vi "PCANTerminal1.vi"() -> ()   [LabVIEW 2020]
uses:
  <userlib>/PCAN-Basic/PCANBasic.lvlib
panel:
  out "x-y":u32
  out "function return 4":u32 format="%x"
  out "function return 3":u32 format="%.0x"
  in  "MessageBuffer":T1(array[cluster])=[{"ID"=828, "MSGTYPE"=0, "LEN"=8, "DATA[0]"=2, "DATA[1]"=0, "DATA[2]"=0, "DATA[3]"=0, "DATA[4]"=0, "DATA[5]"=0, "DATA[6]"=0, "DATA[7]"=0}, {"ID"=860, "MSGTYPE"=0, "LEN"=8, "DATA[0]"=20, "DATA[1]"=0, "DATA[2]"=169, "DATA[3]"=128, "DATA[4]"=74, "DATA[5]"=148, "DATA[6]"=160, "DATA[7]"=9}, {"ID"=917, "MSGTYPE"=0, "LEN"=8, "DATA[0]"=0, "DATA[1]"=0, "DATA[2]"=0, "DATA[3]"=0, "DATA[4]"=0, "DATA[5]"=0, "DATA[6]"=0, "DATA[7]"=0}, {"ID"=1409, "MSGTYPE"=0, "LEN"=8, "DATA[0]"=129, "DATA[1]"=0, "DATA[2]"=0, "DATA[3]"=0, "DATA[4]"=0, "DATA[5]"=0, "DATA[6]"=0, "DATA[7]"=0}, {"ID"=911, "MSGTYPE"=0, "LEN"=8, "DATA[0]"=0, "DATA[1]"=0, "DATA[2]"=8, "DATA[3]"=0, "DATA[4]"=0, "DATA[5]"=0, "DATA[6]"=0, "DATA[7]"=0}] {"ID" format="%.0x"; "DATA[0]" format="%.0x"; "DATA[1]" format="%.0x"; "DATA[2]" format="%.0x"; "DATA[3]" format="%.0x"; "DATA[4]" format="%.0x"; "DATA[5]" format="%.0x"; "DATA[6]" format="%.0x"; "DATA[7]" format="%.0x"}
  out "Exit":bool
  out "function return 2":u32 format="%.0x"
  out "TimestampBuffer out":T2
  out "function return":u32 format="%.0x"
  out "MessageBuffer out":T3 {"ID" format="%.0x"; "DATA[0]" format="%.0x"; "DATA[1]" format="%.0x"; "DATA[2]" format="%.0x"; "DATA[3]" format="%.0x"; "DATA[4]" format="%.0x"; "DATA[5]" format="%.0x"; "DATA[6]" format="%.0x"; "DATA[7]" format="%.0x"}
  in  "停止":bool
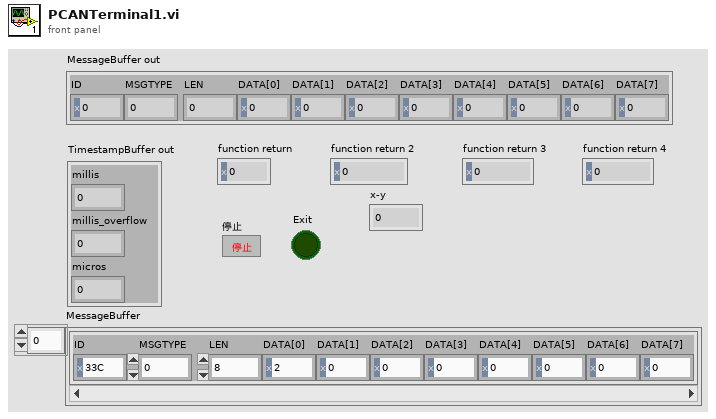
[diagram p1: front panel]
types:
  T1 = cluster{"ID":u32, "MSGTYPE":u8, "LEN":u8, "DATA[0]":u8, "DATA[1]":u8, "DATA[2]":u8, "DATA[3]":u8, "DATA[4]":u8, "DATA[5]":u8, "DATA[6]":u8, "DATA[7]":u8}[]
  T2 = cluster{"millis":u32, "millis_overflow":u16, "micros":u16}
  T3 = cluster{"ID":u32, "MSGTYPE":u8, "LEN":u8, "DATA[0]":u8, "DATA[1]":u8, "DATA[2]":u8, "DATA[3]":u8, "DATA[4]":u8, "DATA[5]":u8, "DATA[6]":u8, "DATA[7]":u8}
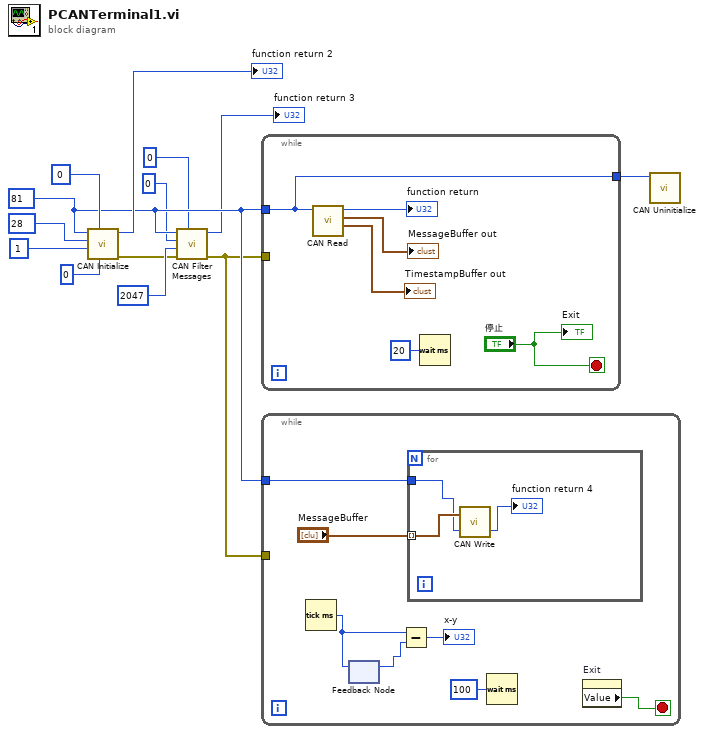
[diagram p0: block diagram]
diagram:
  w7 = u16 81 ("Channel")
  n1 = call <userlib>:"CAN Initialize.vi"("Interrupt"=u16 0, "IOPort"=u32 0, "HwType"=u8 1, "Btr0Btr1"=u16 28, "Channel"=w7) -> ("错误输出"=w2:errorcluster, "function return"=→"function return 2":u32)  [unwired: 5 in]
  n2 = call <userlib>:"CAN Filter Messages.vi"("Mode"=u8 0, "error in (no error)"=w2, "ToID"=u32 2047, "FromID"=u32 0, "Channel"=w7) -> ("error out"=w1:errorcluster, "function return"=→"function return 3":u32)  [unwired: 5 in]
  n3 = while {
    tunnel: w7 -> [w15]
    tunnel: [w15] -> w8
    tunnel: w1 -> [_]
    stop <- "停止" stop-if-true
    n4 = call <userlib>:"CAN Read.vi"("Channel"=w15) -> ("TimestampBuffer out"=→"TimestampBuffer out":T2, "MessageBuffer out"=→"MessageBuffer out":T3, "function return"=→"function return":u32)  [unwired: 7 in, 1 out]
    n5 = Wait (ms)(milliseconds to wait=u32 20 ("等待时间（毫秒）")) -> ()  [unwired: 1 out]
    "Exit" <- "停止"
  }
  n6 = while {
    tunnel: w7 -> [w24]
    tunnel: w1 -> [_]
    stop <- w26 stop-if-true
    n7 = Tick Count (ms)() -> (millisecond timer value=w22:u32)
    n8 = feedback-in #1(w22) -> ()
    n9 = feedback #1() -> (w21:u32)  [unwired: 1 in]
    n10 = Subtract(x=w22, y=w21) -> (x-y=→"x-y":u32)
    n11 = for {
      tunnel: "MessageBuffer" -> [w28] mode=indexing
      tunnel: w24 -> [w27]
      n12 = call <userlib>:"CAN Write.vi"("Channel"=w27, "MessageBuffer"=w28) -> ("function return"=→"function return 4":u32)  [unwired: 1 out]
    }
    n13 = Wait (ms)(milliseconds to wait=u32 100 ("等待时间（毫秒）")) -> ()  [unwired: 1 out]
    n14 = property on="Exit" class="Bool (严格)"() -> ("Value"=w26:bool)  [unwired: 2 in, 2 out]
  }
  n15 = call <userlib>:"CAN Uninitialize.vi"("Channel"=w8) -> ()  [unwired: 10 in, 1 out]
